vi "ILD1420_setup.vi"(5 "Device Name":string) -> (0 "Index":i32, 1 "Measuring range (mm)":u8(ring)=4 items=["10", "25", "50", "100", "200"], 2 "Data Rate Hz":dbl, 3 "Port":string, 4 "Data rate (kHz)":string(combo)="0.25")   [LabVIEW 2022 SP3]
uses:
  Anemometry/Anemometry Sub Vis/Globals/Meas_global.vi
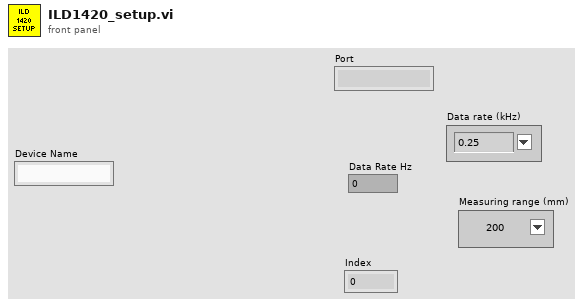
[diagram p1: front panel]
types:
  T1 = typedef "Analysis_info_cluster.ctl" = cluster{"Colour":u32, "Inst type":T2, "Inst name":string, "Symbol":string, "Code name":string, "Extra Info":string, "Inst Array":T3, "Extra Titles":string[], "Extra Values":string[], "U":dbl, "u^2":dbl, "u^3":dbl, "u^4":dbl, "Skew_u":dbl, "Kurt_u":dbl, "Sd Error in Mean":dbl, "% u'/U":dbl, "X":dbl, "Y":dbl, "Z":dbl, "Timescale integral Estimate":dbl, "Sd Error in Variance":dbl, "Calib File":path, "Calib Constants":dbl[], "Output Position":bool, "Stats":enum16{"None", "Basic", "Full"}, "Av Sampling Rate":dbl, "Av No of Samples":dbl, "Total Meas Time (s)":dbl, "ADAM Ch Name":string, "Max value":dbl, "Min value":dbl, "Req Sample Rate Hz":dbl, "Sync Delay Time (s)":dbl, "Ch No":i16, "Device":string, "Use Latest Calib":bool, "Port":string, "Metadata Ch Names":string[], "Metadata Ch Values":string[], "Label":string}
  T2 = typedef "Inst_type.ctl" = enum16{"Raw voltage", "Raw with zero offsetting", "Propeller anemometer", "Pressure Transducer", "Pitot-static tube", "Hot wire", "Cross wire 1", "Cross wire 2", "Generic Linear", "Generic Polynomial", "Generic BackPoly", "Fast FID", "Thermocouple", "Cold wire", "Pulsed Wire", "LDA Vel", "LDA Tran time", "LDA Arr time", "Microphone"}
  T3 = typedef "Instrument_Array.ctl" = enum16{"PWA", "LDA", "Analogue"}
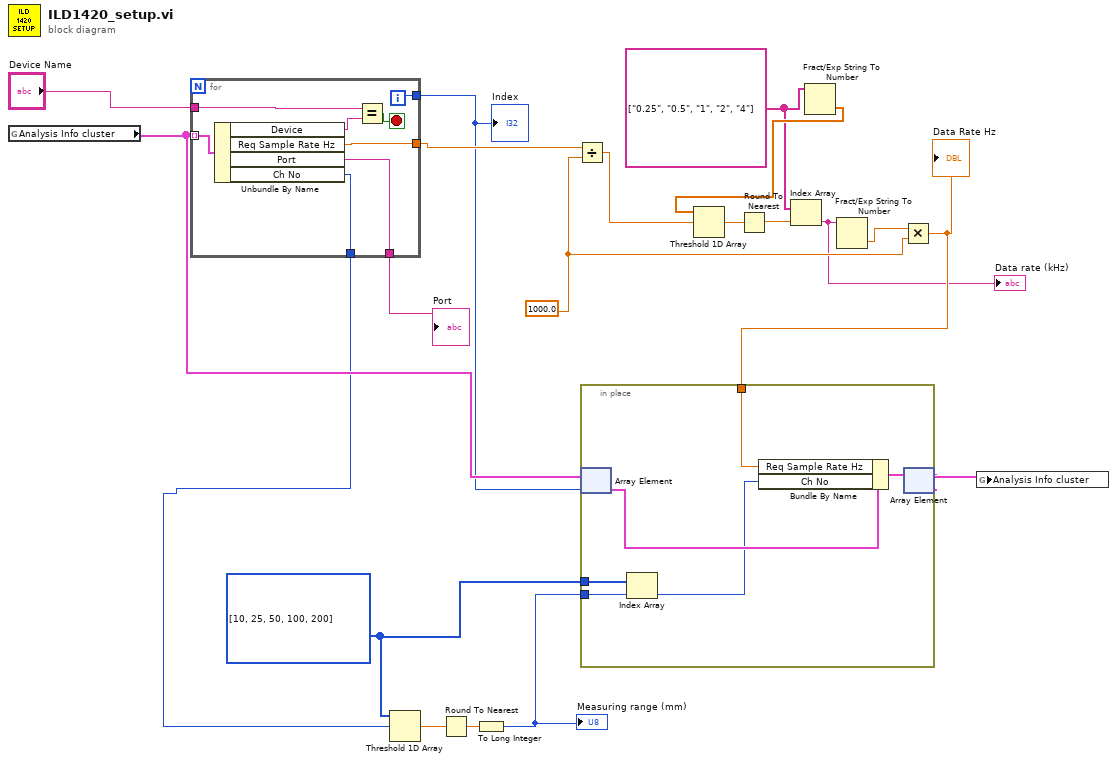
[diagram p0: block diagram]
diagram:
  w10 = i32[] [10, 25, 50, 100, 200]
  w12 = 1000.0 ("y")
  w17 = string[] ["0.25", "0.5", "1", "2", "4"]
  n1 = global read "Meas_global.vi" "Analysis Info cluster"() -> (w7:T1[])
  n2 = for {
    tunnel: w7 -> [w28] mode=indexing
    tunnel: "Device Name" -> [w26]
    tunnel: [w22] -> w5
    tunnel: [w25] -> w13
    tunnel: [w23] -> w4
    tunnel: [w21] -> w3
    i -> [w22]
    stop <- w24 stop-if-true
    n3 = Unbundle By Name(w28) -> ("Device"=w27:string, "Req Sample Rate Hz"=w25:dbl, "Port"=w23:string, "Ch No"=w21:i16)
    n4 = Equal?(x=w26, y=w27) -> (x = y?=w24:bool)
  }
  "Port" <- w4
  "Index" <- w5
  n5 = Threshold 1D Array(2:w3, 3:w10) -> (0:w8:dbl)  [unwired: 1 in]
  n6 = Round To Nearest(number=w8) -> (nearest integer value=w9:dbl)
  n7 = To Long Integer(number=w9) -> (32bit integer=w1:i32)
  "Measuring range (mm)" <- w1
  n8 = Divide(x=w13, y=w12) -> (x/y=w14:dbl)
  n9 = Fract/Exp String To Number(string=w17) -> (number=w18:dbl[])  [unwired: 3 in, 1 out]
  n10 = Threshold 1D Array(2:w14, 3:w18) -> (0:w15:dbl)  [unwired: 1 in]
  n11 = Round To Nearest(number=w15) -> (nearest integer value=w16:dbl)
  n12 = Index Array(array=w17, index=w16) -> (element=w2:string)
  "Data rate (kHz)" <- w2
  n13 = Fract/Exp String To Number(string=w2) -> (number=w19:dbl)  [unwired: 3 in, 1 out]
  n14 = Multiply(x=w19, y=w12) -> (x*y=w6:dbl)
  "Data Rate Hz" <- w6
  n15 = in-place {
    in-place-border: w1 -> [w32]
    in-place-border: w10 -> [w31]
    in-place-border: w6 -> [w29]
    n16 = in-place-array #1(w7, w5) -> (w34:T1)
    n17 = Index Array(array=w31, index=w32) -> (element=w30:i32)
    n18 = Bundle By Name(cluster=w34, "Req Sample Rate Hz"=w29, "Ch No"=w30) -> (w33:T1)
    n19 = in-place-array #1(w33) -> (w11:T1[])  [unwired: 1 out]
  }
  n20 = global write "Meas_global.vi" "Analysis Info cluster"(w11) -> ()
